vi "REPORT_OKNOK_initialize_GUI.vi"(11 "REPORTS_references_in":T1) -> (3 "REPORTS_references_out":T1)   [LabVIEW 2019]
uses:
  FGV/REPORTS_records_display/REPORTS_references.ctl
  GEAR/typedef/REPORT_GEAR_header_data_display.ctl
panel:
  # "GEAR INFO SUMMARY"
  # "GEAR INFO SUMMARY"
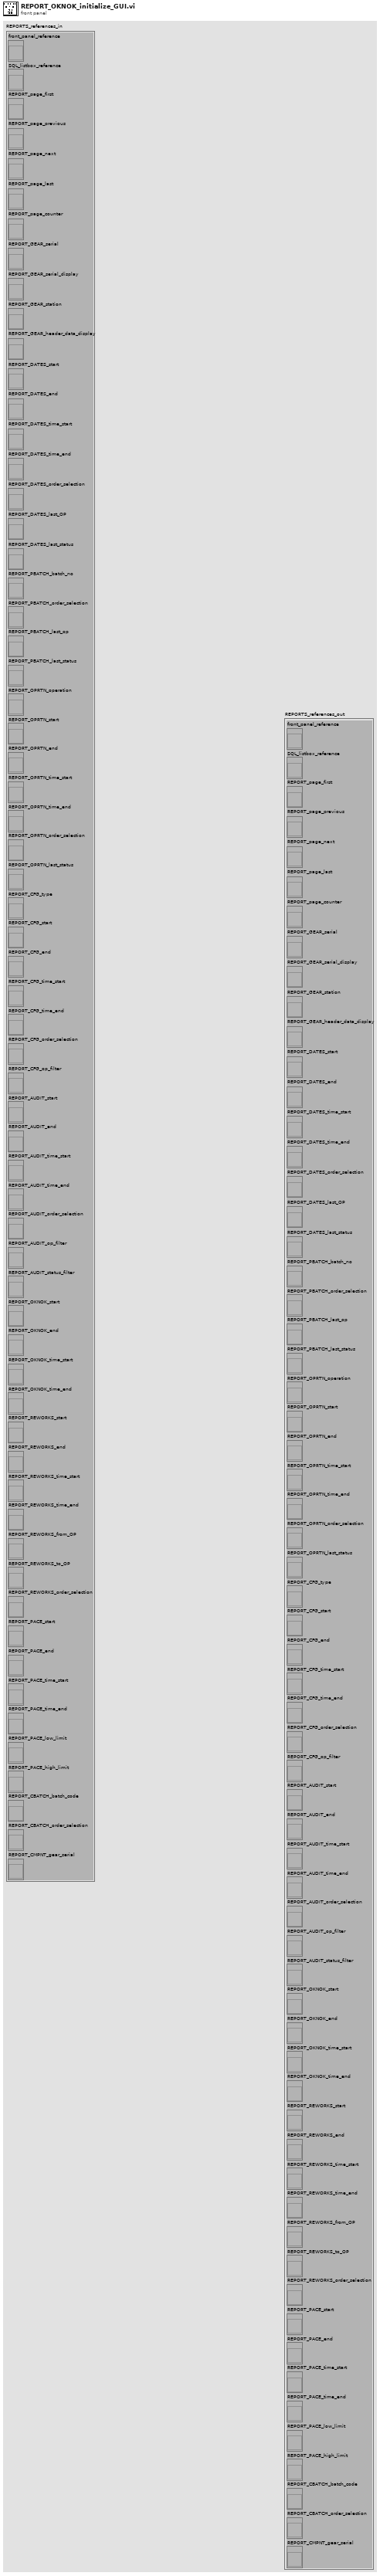
[diagram p1: front panel]
types:
  T1 = typedef "REPORTS_references.ctl" = cluster{"front_panel_reference":refnum<vi>, "SQL_listbox_reference":refnum<vi>, "REPORT_page_first":refnum<vi>, "REPORT_page_previous":refnum<vi>, "REPORT_page_next":refnum<vi>, "REPORT_page_last":refnum<vi>, "REPORT_page_counter":refnum<vi>, "REPORT_GEAR_serial":refnum<vi>, "REPORT_GEAR_serial_display":refnum<vi>, "REPORT_GEAR_station":refnum<vi>, "REPORT_GEAR_header_data_display":refnum<vi>, "REPORT_DATES_start":refnum<vi>, "REPORT_DATES_end":refnum<vi>, "REPORT_DATES_time_start":refnum<vi>, "REPORT_DATES_time_end":refnum<vi>, "REPORT_DATES_order_selection":refnum<vi>, "REPORT_DATES_last_OP":refnum<vi>, "REPORT_DATES_last_status":refnum<vi>, "REPORT_PBATCH_batch_no":refnum<vi>, "REPORT_PBATCH_order_selection":refnum<vi>, "REPORT_PBATCH_last_op":refnum<vi>, "REPORT_PBATCH_last_status":refnum<vi>, "REPORT_OPRTN_operation":refnum<vi>, "REPORT_OPRTN_start":refnum<vi>, "REPORT_OPRTN_end":refnum<vi>, "REPORT_OPRTN_time_start":refnum<vi>, "REPORT_OPRTN_time_end":refnum<vi>, "REPORT_OPRTN_order_selection":refnum<vi>, "REPORT_OPRTN_last_status":refnum<vi>, "REPORT_CFG_type":refnum<vi>, "REPORT_CFG_start":refnum<vi>, "REPORT_CFG_end":refnum<vi>, "REPORT_CFG_time_start":refnum<vi>, "REPORT_CFG_time_end":refnum<vi>, "REPORT_CFG_order_selection":refnum<vi>, "REPORT_CFG_op_filter":refnum<vi>, "REPORT_AUDIT_start":refnum<vi>, "REPORT_AUDIT_end":refnum<vi>, "REPORT_AUDIT_time_start":refnum<vi>, "REPORT_AUDIT_time_end":refnum<vi>, "REPORT_AUDIT_order_selection":refnum<vi>, "REPORT_AUDIT_op_filter":refnum<vi>, "REPORT_AUDIT_status_filter":refnum<vi>, "REPORT_OKNOK_start":refnum<vi>, "REPORT_OKNOK_end":refnum<vi>, "REPORT_OKNOK_time_start":refnum<vi>, "REPORT_OKNOK_time_end":refnum<vi>, "REPORT_REWORKS_start":refnum<vi>, "REPORT_REWORKS_end":refnum<vi>, "REPORT_REWORKS_time_start":refnum<vi>, "REPORT_REWORKS_time_end":refnum<vi>, "REPORT_REWORKS_from_OP":refnum<vi>, "REPORT_REWORKS_to_OP":refnum<vi>, "REPORT_REWORKS_order_selection":refnum<vi>, "REPORT_PACE_start":refnum<vi>, "REPORT_PACE_end":refnum<vi>, "REPORT_PACE_time_start":refnum<vi>, "REPORT_PACE_time_end":refnum<vi>, "REPORT_PACE_low_limit":refnum<vi>, "REPORT_PACE_high_limit":refnum<vi>, "REPORT_CBATCH_batch_code":refnum<vi>, "REPORT_CBATCH_order_selection":refnum<vi>, "REPORT_CMPNT_gear_serial":refnum<vi>}
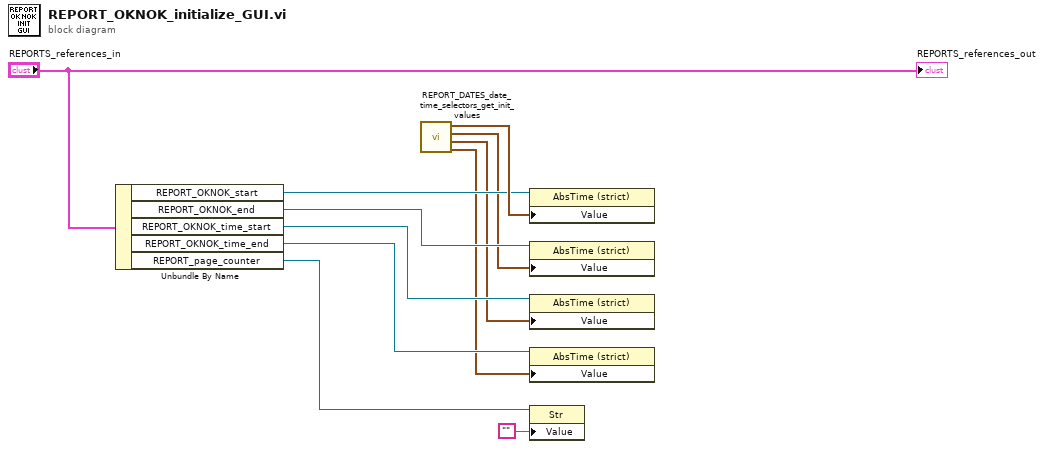
[diagram p0: block diagram]
diagram:
  n1 = Unbundle By Name("REPORTS_references_in") -> ("REPORT_OKNOK_start"=w10:refnum<vi>, "REPORT_OKNOK_end"=w8:refnum<vi>, "REPORT_OKNOK_time_start"=w7:refnum<vi>, "REPORT_OKNOK_time_end"=w6:refnum<vi>, "REPORT_page_counter"=w2:refnum<vi>)
  n2 = call "REPORT_DATES_date_time_selectors_get_init_values.vi"() -> ("time_end"=w3:timestamp, "time_start"=w4:timestamp, "date_end"=w5:timestamp, "date_start"=w11:timestamp)  [unwired: 8 in]
  n3 = property class="AbsTime (strict)"(reference=w10, "Value"=w11) -> ()  [unwired: 1 in, 2 out]
  n4 = property class="AbsTime (strict)"(reference=w8, "Value"=w5) -> ()  [unwired: 1 in, 2 out]
  n5 = property class="AbsTime (strict)"(reference=w7, "Value"=w4) -> ()  [unwired: 1 in, 2 out]
  n6 = property class="AbsTime (strict)"(reference=w6, "Value"=w3) -> ()  [unwired: 1 in, 2 out]
  n7 = property class="Str"(reference=w2, "Value"="") -> ()  [unwired: 1 in, 2 out]
  "REPORTS_references_out" <- "REPORTS_references_in"
